vi "Write Typedef Description.vi"   [LabVIEW 2019, in "JSON-Schema.lvlib"]
uses:
  JSON-Schema.lvlib
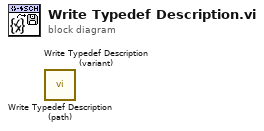
[diagram p0: block diagram]
diagram:
  n1 = call "Write Typedef Description (path).vi"() -> ()  [unwired: 10 in, 2 out]
  n2 = call "Write Typedef Description (variant).vi"() -> ()  [unwired: 10 in, 2 out]
